vi "test_read-nmea-data2.vi"() -> ()   [LabVIEW 2019] (continued)
F9P\t$GNRMC,060930.00,A,3723.60323,N,12656.90330,E,1.432,,250720,,,A,V*10\n\t\n15:09:28.28\tF9P\t$GNVTG,,T,,M,1.432,N,2.653,K,A*3B\n\t\n15:09:28.30\tF9P\t$GNGGA,060930.00,3723.60323,N,12656.90330,E,1,12,0.66,57.5,M,18.5,M,,*78\n\t\n15:09:28.32\tF9P\t$GNGSA,A,3,12,06,19,05,17,09,04,02,,,,,1.21,0.66,1.01,1*02\n\t\n15:09:28.34\tF9P\t$GNGSA,A,3,85,71,84,,,,,,,,,,1.21,0.66,1.01,2*07\n\t\n15:09:28.36\tF9P\t$GNGSA,A,3,36,19,11,04,09,12,,,,,,,1.21,0.66,1.01,3*02\n\t\n15:09:28.38\tF9P\t$GNGSA,A,3,14,11,33,,,,,,,,,,1.21,0.66,1.01,4*03\n\t\n15:09:28.40\tF9P\t$GPGSV,3,1,09,02,54,318,30,04,19,044,21,05,36,246,27,06,65,046,24,1*6E\n\t\n15:09:28.42\tF9P\t$GPGSV,3,2,09,09,45,075,32,12,24,278,25,17,34,153,23,19,53,156,24,1*65\n\t\n15:09:28.44\tF9P\t$GPGSV,3,3,09,25,12,307,23,1*5C\n\t\n15:09:28.46\tF9P\t$GPGSV,3,1,09,02,54,318,,04,19,044,14,05,36,246,18,06,65,046,20,6*64\n\t\n15:09:28.48\tF9P\t$GPGSV,3,2,09,09,45,075,20,12,24,278,16,17,34,153,,19,53,156,,6*66\n\t\n15:09:28.50\tF9P\t$GPGSV,3,3,09,25,12,307,,6*5A\n\t\n15:09:28.52\tF9P\t$GLGSV,2,1,08,69,13,031,,70,73,042,,71,50,204,25,72,03,209,,1*76\n\t\n15:09:28.54\tF9P\t$GLGSV,2,2,08,77,01,327,,84,21,121,12,85,70,063,23,86,35,329,,1*77\n\t\n15:09:28.56\tF9P\t$GLGSV,2,1,08,69,13,031,15,70,73,042,,71,50,204,22,72,03,209,,3*77\n\t\n15:09:28.58\tF9P\t$GLGSV,2,2,08,77,01,327,,84,21,121,17,85,70,063,21,86,35,329,,3*72\n\t\n15:09:28.60\tF9P\t$GAGSV,2,1,08,02,09,298,21,04,65,120,25,09,30,193,17,11,70,356,22,7*70\n\t\n15:09:28.62\tF9P\t$GAGSV,2,2,08,12,41,101,19,19,27,046,10,25,10,250,,36,25,307,28,7*76\n\t\n15:09:28.64\tF9P\t$GAGSV,2,1,08,02,09,298,,04,65,120,26,09,30,193,,11,70,356,19,2*7B\n\t\n15:09:28.66\tF9P\t$GAGSV,2,2,08,12,41,101,,19,27,046,,25,10,250,,36,25,307,23,2*71\n\t\n15:09:28.68\tF9P\t$GBGSV,1,1,03,11,51,130,12,14,86,148,17,33,59,218,21,1*44\n\t\n15:09:28.70\tF9P\t$GBGSV,1,1,04,08,,,21,11,51,130,23,14,86,148,30,33,59,218,,3*4E\n\t\n15:09:28.72\tF9P\t$GNGLL,3723.60323,N,12656.90330,E,060930.00,A,A*75\n\t\n15:09:28.74\tF9P\t\t\n15:09:28.76\tF9P\t\t\n15:09:28.78\tF9P\t\t\n15:09:28.80\tF9P\t\t\n15:09:28.82\tF9P\t\t\n15:09:28.84\tF9P\t\t\n15:09:28.86\tF9P\t\t\n15:09:28.88\tF9P\t\t\n15:09:28.90\tF9P\t\t\n15:09:28.92\tF9P\t\t\n15:09:28.94\tF9P\t\t\n15:09:28.96\tF9P\t\t\n15:09:28.98\tF9P\t\t\n15:09:29.00\tF9P\t\t\n15:09:29.02\tF9P\t\t\n15:09:29.04\tF9P\t\t\n15:09:29.06\tF9P\t\t\n15:09:29.08\tF9P\t\t\n15:09:29.10\tF9P\t\t\n15:09:29.12\tF9P\t\t\n15:09:29.14\tF9P\t\t\n15:09:29.16\tF9P\t\t\n15:09:29.18\tF9P\t\t\n15:09:29.20\tF9P\t\t\n15:09:29.22\tF9P\t\t\n15:09:29.24\tF9P\t$GNRMC,060931.00,A,3723.60267,N,12656.90271,E,2.484,237.32,250720,,,A,V*03\n\t\n15:09:29.26\tF9P\t$GNVTG,237.32,T,,M,2.484,N,4.600,K,A*2C\n\t\n15:09:29.28\tF9P\t$GNGGA,060931.00,3723.60267,N,12656.90271,E,1,12,0.67,56.1,M,18.5,M,,*78\n\t\n15:09:29.30\tF9P\t$GNGSA,A,3,12,06,19,05,17,09,04,02,,,,,1.23,0.67,1.03,1*03\n\t\n15:09:29.32\tF9P\t$GNGSA,A,3,85,71,84,,,,,,,,,,1.23,0.67,1.03,2*06\n\t\n15:09:29.34\tF9P\t$GNGSA,A,3,36,19,11,04,09,12,,,,,,,1.23,0.67,1.03,3*03\n\t\n15:09:29.36\tF9P\t$GNGSA,A,3,14,11,33,,,,,,,,,,1.23,0.67,1.03,4*02\n\t\n15:09:29.38\tF9P\t$GPGSV,3,1,09,02,54,318,24,04,19,044,19,05,36,246,33,06,65,046,23,1*62\n\t\n15:09:29.40\tF9P\t$GPGSV,3,2,09,09,45,075,24,12,24,278,24,17,34,153,30,19,53,156,23,1*66\n\t\n15:09:29.42\tF9P\t$GPGSV,3,3,09,25,12,307,23,1*5C\n\t\n15:09:29.44\tF9P\t$GPGSV,3,1,09,02,54,318,,04,19,044,14,05,36,246,16,06,65,046,21,6*6B\n\t\n15:09:29.46\tF9P\t$GPGSV,3,2,09,09,45,075,18,12,24,278,17,17,34,153,,19,53,156,,6*6C\n\t\n15:09:29.48\tF9P\t$GPGSV,3,3,09,25,12,307,,6*5A\n\t\n15:09:29.50\tF9P\t$GLGSV,2,1,08,69,13,031,,70,73,042,,71,50,204,32,72,03,209,,1*70\n\t\n15:09:29.52\tF9P\t$GLGSV,2,2,08,77,01,327,,84,21,121,13,85,70,063,24,86,35,329,,1*71\n\t\n15:09:29.54\tF9P\t$GLGSV,2,1,08,69,13,031,,70,73,042,,71,50,204,23,72,03,209,,3*72\n\t\n15:09:29.56\tF9P\t$GLGSV,2,2,08,77,01,327,,84,21,121,16,85,70,063,20,86,35,329,,3*72\n\t\n15:09:29.58\tF9P\t$GAGSV,2,1,08,02,09,298,17,04,65,120,24,09,30,193,16,11,70,356,23,7*74\n\t\n15:09:29.60\tF9P\t$GAGSV,2,2,08,12,41,101,17,19,27,046,14,25,10,250,,36,25,307,32,7*77\n\t\n15:09:29.62\tF9P\t$GAGSV,2,1,08,02,09,298,,04,65,120,27,09,30,193,,11,70,356,19,2*7A\n\t\n15:09:29.64\tF9P\t$GAGSV,2,2,08,12,41,101,,19,27,046,,25,10,250,,36,25,307,23,2*71\n\t\n15:09:29.66\tF9P\t$GBGSV,1,1,03,11,51,130,07,14,86,148,10,33,59,218,17,1*42\n\t\n15:09:29.68\tF9P\t$GBGSV,1,1,04,08,,,20,11,51,130,21,14,86,148,29,33,59,218,,3*45\n\t\n15:09:29.70\tF9P\t$GNGLL,3723.60267,N,12656.90271,E,060931.00,A,A*71\n\t\n15:09:29.72\tF9P\t\t\n15:09:29.74\tF9P\t\t\n15:09:29.76\tF9P\t\t\n15:09:29.78\tF9P\t\t\n15:09:29.80\tF9P\t\t\n15:09:29.82\tF9P\t\t\n15:09:29.84\tF9P\t\t\n15:09:29.86\tF9P\t\t\n15:09:29.88\tF9P\t\t\n15:09:29.90\tF9P\t\t\n15:09:29.92\tF9P\t\t\n15:09:29.94\tF9P\t\t\n15:09:29.96\tF9P\t\t\n15:09:29.98\tF9P\t\t\n15:09:30.00\tF9P\t\t\n15:09:30.02\tF9P\t\t\n15:09:30.05\tF9P\t\t\n15:09:30.07\tF9P\t\t\n15:09:30.09\tF9P\t\t\n15:09:30.11\tF9P\t\t\n15:09:30.13\tF9P\t\t\n15:09:30.15\tF9P\t\t\n15:09:30.17\tF9P\t\t\n15:09:30.19\tF9P\t\t\n15:09:30.21\tF9P\t\t\n15:09:30.23\tF9P\t\t\n15:09:30.25\tF9P\t$GNRMC,060932.00,A,3723.60237,N,12656.90214,E,1.383,237.05,250720,,,A,V*01\n\t\n15:09:30.27\tF9P\t$GNVTG,237.05,T,,M,1.383,N,2.562,K,A*2A\n\t\n15:09:30.29\tF9P\t$GNGGA,060932.00,3723.60237,N,12656.90214,E,1,12,0.67,55.8,M,18.5,M,,*77\n\t\n15:09:30.31\tF9P\t$GNGSA,A,3,12,06,19,05,17,09,04,02,,,,,1.23,0.67,1.03,1*03\n\t\n15:09:30.33\tF9P\t$GNGSA,A,3,85,71,84,,,,,,,,,,1.23,0.67,1.03,2*06\n\t\n15:09:30.35\tF9P\t$GNGSA,A,3,36,19,11,04,09,12,,,,,,,1.23,0.67,1.03,3*03\n\t\n15:09:30.37\tF9P\t$GNGSA,A,3,14,11,,,,,,,,,,,1.23,0.67,1.03,4*02\n\t\n15:09:30.39\tF9P\t$GPGSV,3,1,09,02,54,318,31,04,19,044,17,05,36,246,29,06,65,046,29,1*69\n\t\n15:09:30.41\tF9P\t$GPGSV,3,2,09,09,45,075,28,12,24,278,23,17,34,153,24,19,53,156,33,1*69\n\t\n15:09:30.43\tF9P\t$GPGSV,3,3,09,25,12,307,24,1*5B\n\t\n15:09:30.45\tF9P\t$GPGSV,3,1,09,02,54,318,,04,19,044,12,05,36,246,17,06,65,046,20,6*6D\n\t\n15:09:30.47\tF9P\t$GPGSV,3,2,09,09,45,075,17,12,24,278,16,17,34,153,,19,53,156,,6*62\n\t\n15:09:30.49\tF9P\t$GPGSV,3,3,09,25,12,307,,6*5A\n\t\n15:09:30.51\tF9P\t$GLGSV,2,1,08,69,13,031,,70,73,042,,71,50,204,30,72,03,209,,1*72\n\t\n15:09:30.53\tF9P\t$GLGSV,2,2,08,77,01,327,,84,21,121,12,85,70,063,30,86,35,329,,1*75\n\t\n15:09:30.55\tF9P\t$GLGSV,2,1,08,69,13,031,,70,73,042,,71,50,204,24,72,03,209,,3*75\n\t\n15:09:30.57\tF9P\t$GLGSV,2,2,08,77,01,327,,84,21,121,17,85,70,063,19,86,35,329,,3*79\n\t\n15:09:30.59\tF9P\t$GAGSV,2,1,08,02,09,298,16,04,65,120,24,09,30,193,16,11,70,356,23,7*75\n\t\n15:09:30.61\tF9P\t$GAGSV,2,2,08,12,41,101,16,19,27,046,13,25,10,250,,36,25,307,29,7*7B\n\t\n15:09:30.63\tF9P\t$GAGSV,2,1,08,02,09,298,,04,65,120,27,09,30,193,,11,70,356,21,2*71\n\t\n15:09:30.65\tF9P\t$GAGSV,2,2,08,12,41,101,,19,27,046,,25,10,250,,36,25,307,25,2*77\n\t\n15:09:30.67\tF9P\t$GBGSV,1,1,03,11,51,130,,14,86,148,07,33,59,218,,1*45\n\t\n15:09:30.69\tF9P\t$GBGSV,1,1,04,08,,,18,11,51,130,21,14,86,148,32,33,59,218,,3*44\n\t\n15:09:30.71\tF9P\t$GNGLL,3723.60237,N,12656.90214,E,060932.00,A,A*74\n\t\n15:09:30.73\tF9P\t\t\n15:09:30.75\tF9P\t\t\n15:09:30.77\tF9P\t\t\n15:09:30.79\tF9P\t\t\n15:09:30.81\tF9P\t\t\n15:09:30.83\tF9P\t\t\n15:09:30.85\tF9P\t\t\n15:09:30.87\tF9P\t\t\n15:09:30.89\tF9P\t\t\n15:09:30.91\tF9P\t\t\n15:09:30.93\tF9P\t\t\n15:09:30.95\tF9P\t\t\n15:09:30.97\tF9P\t\t\n15:09:30.99\tF9P\t\t\n15:09:31.01\tF9P\t\t\n15:09:31.03\tF9P\t\t\n15:09:31.05\tF9P\t\t\n15:09:31.07\tF9P\t\t\n15:09:31.09\tF9P\t\t\n15:09:31.11\tF9P\t\t\n15:09:31.13\tF9P\t\t\n15:09:31.15\tF9P\t\t\n15:09:31.17\tF9P\t\t\n15:09:31.19\tF9P\t\t\n15:09:31.21\tF9P\t\t\n15:09:31.23\tF9P\t\t\n15:09:31.25\tF9P\t$GNRMC,060933.00,A,3723.60178,N,12656.90204,E,1.526,218.15,250720,,,A,V*0C\n\t\n15:09:31.27\tF9P\t$GNVTG,218.15,T,,M,1.526,N,2.826,K,A*22\n\t\n15:09:31.29\tF9P\t$GNGGA,060933.00,3723.60178,N,12656.90204,E,1,12,0.69,54.6,M,18.5,M,,*7E\n\t\n15:09:31.31\tF9P\t$GNGSA,A,3,12,06,19,05,17,09,02,,,,,,1.30,0.69,1.11,1*08\n\t\n15:09:31.33\tF9P\t$GNGSA,A,3,85,71,84,,,,,,,,,,1.30,0.69,1.11,2*09\n\t\n15:09:31.35\tF9P\t$GNGSA,A,3,36,19,11,04,09,12,,,,,,,1.30,0.69,1.11,3*0C\n\t\n15:09:31.37\tF9P\t$GNGSA,A,3,14,11,,,,,,,,,,,1.30,0.69,1.11,4*0D\n\t\n15:09:31.39\tF9P\t$GPGSV,3,1,09,02,54,318,30,04,19,044,,05,36,246,27,06,65,046,27,1*6E\n\t\n15:09:31.41\tF9P\t$GPGSV,3,2,09,09,45,075,28,12,24,278,27,17,34,153,30,19,53,156,32,1*69\n\t\n15:09:31.43\tF9P\t$GPGSV,3,3,09,25,12,307,27,1*58\n\t\n15:09:31.45\tF9P\t$GPGSV,3,1,09,02,54,318,,04,19,044,13,05,36,246,19,06,65,046,20,6*62\n\t\n15:09:31.47\tF9P\t$GPGSV,3,2,09,09,45,075,17,12,24,278,15,17,34,153,,19,53,156,,6*61\n\t\n15:09:31.49\tF9P\t$GPGSV,3,3,09,25,12,307,,6*5A\n\t\n15:09:31.51\tF9P\t$GLGSV,2,1,08,69,13,031,,70,73,042,,71,50,204,29,72,03,209,,1*7A\n\t\n15:09:31.53\tF9P\t$GLGSV,2,2,08,77,01,327,,84,21,121,12,85,70,063,30,86,35,329,,1*75\n\t\n15:09:31.55\tF9P\t$GLGSV,2,1,08,69,13,031,,70,73,042,,71,50,204,25,72,03,209,,3*74\n\t\n15:09:31.57\tF9P\t$GLGSV,2,2,08,77,01,327,,84,21,121,19,85,70,063,19,86,35,329,,3*77\n\t\n15:09:31.59\tF9P\t$GAGSV,2,1,08,02,09,298,15,04,65,120,29,09,30,193,14,11,70,356,22,7*78\n\t\n15:09:31.61\tF9P\t$GAGSV,2,2,08,12,41,101,17,19,27,046,11,25,10,250,,36,25,307,32,7*72\n\t\n15:09:31.63\tF9P\t$GAGSV,2,1,08,02,09,298,,04,65,120,27,09,30,193,,11,70,356,22,2*72\n\t\n15:09:31.65\tF9P\t$GAGSV,2,2,08,12,41,101,,19,27,046,,25,10,250,,36,25,307,30,2*73\n\t\n15:09:31.67\tF9P\t$GBGSV,1,1,04,07,,,21,11,51,130,,14,86,148,18,33,59,218,25,1*4F\n\t\n15:09:31.69\tF9P\t$GBGSV,1,1,04,08,,,27,11,51,130,21,14,86,148,32,33,59,218,,3*48\n\t\n15:09:31.71\tF9P\t$GNGLL,3723.60178,N,12656.90204,E,060933.00,A,A*7C\n\t\n15:09:31.73\tF9P\t\t\n15:09:31.75\tF9P\t\t\n15:09:31.77\tF9P\t\t\n15:09:31.79\tF9P\t\t\n15:09:31.81\tF9P\t\t\n15:09:31.83\tF9P\t\t\n15:09:31.85\tF9P\t\t\n15:09:31.87\tF9P\t\t\n15:09:31.89\tF9P\t\t\n15:09:31.91\tF9P\t\t\n15:09:31.93\tF9P\t\t\n15:09:31.95\tF9P\t\t\n15:09:31.97\tF9P\t\t\n15:09:31.99\tF9P\t\t\n15:09:32.01\tF9P\t\t\n15:09:32.03\tF9P\t\t\n15:09:32.05\tF9P\t\t\n15:09:32.07\tF9P\t\t\n15:09:32.09\tF9P\t\t\n15:09:32.11\tF9P\t\t\n15:09:32.13\tF9P\t\t\n15:09:32.15\tF9P\t\t\n15:09:32.17\tF9P\t\t\n15:09:32.19\tF9P\t\t\n15:09:32.21\tF9P\t\t\n15:09:32.23\tF9P\t\t\n15:09:32.25\tF9P\t$GNRMC,060934.00,A,3723.60110,N,12656.90170,E,1.480,224.53,250720,,,A,V*05\n\t\n15:09:32.27\tF9P\t$GNVTG,224.53,T,,M,1.480,N,2.741,K,A*2C\n\t\n15:09:32.29\tF9P\t$GNGGA,060934.00,3723.60110,N,12656.90170,E,1,12,0.68,54.6,M,18.5,M,,*76\n\t\n15:09:32.31\tF9P\t$GNGSA,A,3,12,06,19,05,17,09,04,02,,,,,1.31,0.68,1.12,1*0F\n\t\n15:09:32.33\tF9P\t$GNGSA,A,3,85,71,84,,,,,,,,,,1.31,0.68,1.12,2*0A\n\t\n15:09:32.35\tF9P\t$GNGSA,A,3,36,19,11,04,09,12,,,,,,,1.31,0.68,1.12,3*0F\n\t\n15:09:32.37\tF9P\t$GNGSA,A,3,14,11,33,,,,,,,,,,1.31,0.68,1.12,4*0E\n\t\n15:09:32.39\tF9P\t$GPGSV,3,1,09,02,54,318,34,04,19,044,20,05,36,246,31,06,65,046,27,1*6F\n\t\n15:09:32.41\tF9P\t$GPGSV,3,2,09,09,45,075,32,12,24,278,26,17,34,153,32,19,53,156,27,1*65\n\t\n15:09:32.43\tF9P\t$GPGSV,3,3,09,25,12,307,26,1*59\n\t\n15:09:32.45\tF9P\t$GPGSV,3,1,09,02,54,318,,04,19,044,12,05,36,246,20,06,65,046,21,6*68\n\t\n15:09:32.47\tF9P\t$GPGSV,3,2,09,09,45,075,18,12,24,278,15,17,34,153,,19,53,156,,6*6E\n\t\n15:09:32.49\tF9P\t$GPGSV,3,3,09,25,12,307,,6*5A\n\t\n15:09:32.51\tF9P\t$GLGSV,2,1,08,69,13,031,,70,73,042,,71,50,204,33,72,03,209,,1*71\n\t\n15:09:32.53\tF9P\t$GLGSV,2,2,08,77,01,327,,84,21,121,12,85,70,063,29,86,35,329,,1*7D\n\t\n15:09:32.55\tF9P\t$GLGSV,2,1,08,69,13,031,,70,73,042,,71,50,204,25,72,03,209,,3*74\n\t\n15:09:32.57\tF9P\t$GLGSV,2,2,08,77,01,327,,84,21,121,18,85,70,063,19,86,35,329,,3*76\n\t\n15:09:32.59\tF9P\t$GAGSV,2,1,08,02,09,298,15,04,65,120,30,09,30,193,16,11,70,356,22,7*72\n\t\n15:09:32.61\tF9P\t$GAGSV,2,2,08,12,41,101,17,19,27,046,11,25,10,250,,36,25,307,26,7*77\n\t\n15:09:32.63\tF9P\t$GAGSV,2,1,08,02,09,298,,04,65,120,25,09,30,193,,11,70,356,22,2*70\n\t\n15:09:32.65\tF9P\t$GAGSV,2,2,08,12,41,101,,19,27,046,,25,10,250,,36,25,307,23,2*71\n\t\n15:09:32.67\tF9P\t$GBGSV,2,1,06,06,,,23,07,,,28,08,,,27,11,51,130,12,1*41\n\t\n15:09:32.69\tF9P\t$GBGSV,2,2,06,14,86,148,18,33,59,218,33,1*78\n\t\n15:09:32.71\tF9P\t$GBGSV,1,1,04,08,,,27,11,51,130,21,14,86,148,26,33,59,218,,3*4D\n\t\n15:09:32.73\tF9P\t$GNGLL,3723.60110,N,12656.90170,E,060934.00,A,A*75\n\t\n15:09:32.75\tF9P\t\t\n15:09:32.77\tF9P\t\t\n15:09:32.79\tF9P\t\t\n15:09:32.81\tF9P\t\t\n15:09:32.83\tF9P\t\t\n15:09:32.85\tF9P\t\t\n15:09:32.87\tF9P\t\t\n15:09:32.89\tF9P\t\t\n15:09:32.91\tF9P\t\t\n15:09:32.93\tF9P\t\t\n15:09:32.95\tF9P\t\t\n15:09:32.97\tF9P\t\t\n15:09:32.99\tF9P\t\t\n15:09:33.01\tF9P\t\t\n15:09:33.03\tF9P\t\t\n15:09:33.05\tF9P\t\t\n15:09:33.07\tF9P\t\t\n15:09:33.09\tF9P\t\t\n15:09:33.11\tF9P\t\t\n15:09:33.13\tF9P\t\t\n15:09:33.15\tF9P\t\t\n15:09:33.17\tF9P\t\t\n15:09:33.19\tF9P\t\t\n15:09:33.21\tF9P\t\t\n15:09:33.23\tF9P\t\t\n15:09:33.25\tF9P\t$GNRMC,060935.00,A,3723.60013,N,12656.90147,E,2.238,224.68,250720,,,A,V*0C\n\t\n15:09:33.27\tF9P\t$GNVTG,224.68,T,,M,2.238,N,4.145,K,A*26\n\t\n15:09:33.29\tF9P\t$GNGGA,060935.00,3723.60013,N,12656.90147,E,1,12,0.64,52.8,M,18.5,M,,*75\n\t\n15:09:33.31\tF9P\t$GNGSA,A,3,12,06,19,05,17,09,04,02,,,,,1.19,0.64,1.00,1*0A\n\t\n15:09:33.33\tF9P\t$GNGSA,A,3,85,71,84,,,,,,,,,,1.19,0.64,1.00,2*0F\n\t\n15:09:33.35\tF9P\t$GNGSA,A,3,36,19,11,04,09,12,,,,,,,1.19,0.64,1.00,3*0A\n\t\n15:09:33.37\tF9P\t$GNGSA,A,3,14,11,33,,,,,,,,,,1.19,0.64,1.00,4*0B\n\t\n15:09:33.39\tF9P\t$GPGSV,3,1,09,02,54,318,28,04,19,044,20,05,36,246,28,06,65,046,32,1*6E\n\t\n15:09:33.41\tF9P\t$GPGSV,3,2,09,09,45,075,32,12,24,278,24,17,34,153,34,19,53,156,34,1*63\n\t\n15:09:33.43\tF9P\t$GPGSV,3,3,09,25,12,307,25,1*5A\n\t\n15:09:33.45\tF9P\t$GPGSV,3,1,09,02,54,318,,04,19,044,12,05,36,246,19,06,65,046,21,6*62\n\t\n15:09:33.47\tF9P\t$GPGSV,3,2,09,09,45,075,21,12,24,278,13,17,34,153,21,19,53,156,,6*61\n\t\n15:09:33.49\tF9P\t$GPGSV,3,3,09,25,12,307,,6*5A\n\t\n15:09:33.51\tF9P\t$GLGSV,2,1,08,69,13,031,,70,73,042,,71,50,204,29,72,03,209,,1*7A\n\t\n15:09:33.53\tF9P\t$GLGSV,2,2,08,77,01,327,,84,21,121,10,85,70,063,27,86,35,329,,1*71\n\t\n15:09:33.55\tF9P\t$GLGSV,2,1,08,69,13,031,,70,73,042,,71,50,204,26,72,03,209,,3*77\n\t\n15:09:33.57\tF9P\t$GLGSV,2,2,08,77,01,327,,84,21,121,19,85,70,063,19,86,35,329,,3*77\n\t\n15:09:33.59\tF9P\t$GAGSV,2,1,08,02,09,298,12,04,66,119,28,09,30,193,16,11,70,356,23,7*74\n\t\n15:09:33.61\tF9P\t$GAGSV,2,2,08,12,41,101,17,19,27,046,10,25,10,250,,36,25,307,29,7*79\n\t\n15:09:33.63\tF9P\t$GAGSV,2,1,08,02,09,298,,04,66,119,24,09,30,193,,11,70,356,21,2*7B\n\t\n15:09:33.65\tF9P\t$GAGSV,2,2,08,12,41,101,,19,27,046,,25,10,250,,36,25,307,22,2*70\n\t\n15:09:33.67\tF9P\t$GBGSV,2,1,06,06,,,25,07,,,25,08,,,25,11,51,130,13,1*49\n\t\n15:09:33.69\tF9P\t$GBGSV,2,2,06,14,86,148,27,33,59,218,25,1*73\n\t\n15:09:33.71\tF9P\t$GBGSV,1,1,04,08,,,26,11,51,130,22,14,86,148,31,33,59,218,,3*49\n\t\n15:09:33.73\tF9P\t$GNGLL,3723.60013,N,12656.90147,E,060935.00,A,A*72\n\t\n15:09:33.75\tF9P\t\t\n15:09:33.77\tF9P\t\t\n15:09:33.79\tF9P\t\t\n15:09:33.81\tF9P\t\t\n15:09:33.83\tF9P\t\t\n15:09:33.85\tF9P\t\t\n15:09:33.87\tF9P\t\t\n15:09:33.89\tF9P\t\t\n15:09:33.91\tF9P\t\t\n15:09:33.93\tF9P\t\t\n15:09:33.95\tF9P\t\t\n15:09:33.97\tF9P\t\t\n15:09:33.99\tF9P\t\t\n15:09:34.01\tF9P\t\t\n15:09:34.03\tF9P\t\t\n15:09:34.05\tF9P\t\t\n15:09:34.07\tF9P\t\t\n15:09:34.09\tF9P\t\t\n15:09:34.11\tF9P\t\t\n15:09:34.13\tF9P\t\t\n15:09:34.15\tF9P\t\t\n15:09:34.17\tF9P\t\t\n15:09:34.19\tF9P\t\t\n15:09:34.21\tF9P\t\t\n15:09:34.23\tF9P\t\t\n15:09:34.25\tF9P\t$GNRMC,060936.00,A,3723.59866,N,12656.90154,E,2.355,237.67,250720,,,A,V*0A\n\t\n15:09:34.27\tF9P\t$GNVTG,237.67,T,,M,2.355,N,4.361,K,A*25\n\t\n15:09:34.29\tF9P\t$GNGGA,060936.00,3723.59866,N,12656.90154,E,1,12,0.64,49.6,M,18.5,M,,*70\n\t\n15:09:34.31\tF9P\t$GNGSA,A,3,12,06,19,05,17,09,04,02,,,,,1.19,0.64,1.00,1*0A\n\t\n15:09:34.33\tF9P\t$GNGSA,A,3,85,71,84,,,,,,,,,,1.19,0.64,1.00,2*0F\n\t\n15:09:34.35\tF9P\t$GNGSA,A,3,36,19,11,04,09,12,,,,,,,1.19,0.64,1.00,3*0A\n\t\n15:09:34.37\tF9P\t$GNGSA,A,3,14,11,33,,,,,,,,,,1.19,0.64,1.00,4*0B\n\t\n15:09:34.39\tF9P\t$GPGSV,3,1,09,02,54,318,27,04,19,044,17,05,36,246,32,06,65,046,31,1*6D\n\t\n15:09:34.41\tF9P\t$GPGSV,3,2,09,09,45,075,35,12,24,278,21,17,34,153,39,19,53,156,31,1*69\n\t\n15:09:34.43\tF9P\t$GPGSV,3,3,09,25,12,307,22,1*5D\n\t\n15:09:34.45\tF9P\t$GPGSV,3,1,09,02,54,318,,04,19,044,13,05,36,246,18,06,65,046,22,6*61\n\t\n15:09:34.47\tF9P\t$GPGSV,3,2,09,09,45,075,22,12,24,278,13,17,34,153,22,19,53,156,,6*61\n\t\n15:09:34.49\tF9P\t$GPGSV,3,3,09,25,12,307,,6*5A\n\t\n15:09:34.51\tF9P\t$GLGSV,2,1,08,69,13,031,,70,73,042,,71,50,204,28,72,03,209,,1*7B\n\t\n15:09:34.53\tF9P\t$GLGSV,2,2,08,77,01,327,,84,21,121,09,85,70,063,26,86,35,329,,1*78\n\t\n15:09:34.55\tF9P\t$GLGSV,2,1,08,69,13,031,,70,73,042,,71,50,204,24,72,03,209,,3*75\n\t\n15:09:34.57\tF9P\t$GLGSV,2,2,08,77,01,327,,84,21,121,18,85,70,063,19,86,35,329,,3*76\n\t\n15:09:34.59\tF9P\t$GAGSV,2,1,08,02,09,298,12,04,66,119,32,09,30,193,20,11,70,356,24,7*7D\n\t\n15:09:34.61\tF9P\t$GAGSV,2,2,08,12,41,101,16,19,27,046,09,25,10,250,,36,25,307,29,7*70\n\t\n15:09:34.63\tF9P\t$GAGSV,2,1,08,02,09,298,,04,66,119,24,09,30,193,22,11,70,356,19,2*70\n\t\n15:09:34.65\tF9P\t$GAGSV,2,2,08,12,41,101,,19,27,046,,25,10,250,,36,25,307,23,2*71\n\t\n15:09:34.67\tF9P\t$GBGSV,1,1,03,11,51,130,15,14,86,148,28,33,59,218,25,1*4B\n\t\n15:09:34.69\tF9P\t$GBGSV,1,1,04,08,,,24,11,51,130,22,14,86,148,30,33,59,218,,3*4A\n\t\n15:09:34.71\tF9P\t$GNGLL,3723.59866,N,12656.90154,E,060936.00,A,A*73\n\t\n15:09:34.73\tF9P\t\t\n15:09:34.75\tF9P\t\t\n15:09:34.77\tF9P\t\t\n15:09:34.79\tF9P\t\t\n15:09:34.81\tF9P\t\t\n15:09:34.83\tF9P\t\t\n15:09:34.85\tF9P\t\t\n15:09:34.87\tF9P\t\t\n15:09:34.89\tF9P\t\t\n15:09:34.91\tF9P\t\t\n15:09:34.93\tF9P\t\t\n15:09:34.95\tF9P\t\t\n15:09:34.97\tF9P\t\t\n15:09:34.99\tF9P\t\t\n15:09:35.01\tF9P\t\t\n15:09:35.03\tF9P\t\t\n15:09:35.05\tF9P\t\t\n15:09:35.07\tF9P\t\t\n15:09:35.09\tF9P\t\t\n15:09:35.11\tF9P\t\t\n15:09:35.13\tF9P\t\t\n15:09:35.15\tF9P\t\t\n15:09:35.17\tF9P\t\t\n15:09:35.19\tF9P\t\t\n15:09:35.21\tF9P\t\t\n15:09:35.23\tF9P\t\t\n15:09:35.25\tF9P\t$GNRMC,060937.00,A,3723.59722,N,12656.90157,E,2.229,233.59,250720,,,A,V*04\n\t\n15:09:35.27\tF9P\t$GNVTG,233.59,T,,M,2.229,N,4.128,K,A*29\n\t\n15:09:35.29\tF9P\t$GNGGA,060937.00,3723.59722,N,12656.90157,E,1,12,0.67,47.2,M,18.5,M,,*74\n\t\n15:09:35.31\tF9P\t$GNGSA,A,3,12,06,19,05,17,09,04,02,,,,,1.29,0.67,1.10,1*0B\n\t\n15:09:35.33\tF9P\t$GNGSA,A,3,85,71,84,,,,,,,,,,1.29,0.67,1.10,2*0E\n\t\n15:09:35.35\tF9P\t$GNGSA,A,3,36,19,11,04,09,12,,,,,,,1.29,0.67,1.10,3*0B\n\t\n15:09:35.37\tF9P\t$GNGSA,A,3,14,11,33,,,,,,,,,,1.29,0.67,1.10,4*0A\n\t\n15:09:35.39\tF9P\t$GPGSV,3,1,09,02,54,318,28,04,19,044,17,05,36,246,28,06,65,046,29,1*60\n\t\n15:09:35.41\tF9P\t$GPGSV,3,2,09,09,45,075,30,12,24,278,20,17,34,153,38,19,53,156,32,1*6F\n\t\n15:09:35.43\tF9P\t$GPGSV,3,3,09,25,12,307,22,1*5D\n\t\n15:09:35.45\tF9P\t$GPGSV,3,1,09,02,54,318,,04,19,044,10,05,36,246,20,06,65,046,24,6*6F\n\t\n15:09:35.47\tF9P\t$GPGSV,3,2,09,09,45,075,22,12,24,278,,17,34,153,24,19,53,156,,6*65\n\t\n15:09:35.49\tF9P\t$GPGSV,3,3,09,25,12,307,,6*5A\n\t\n15:09:35.51\tF9P\t$GLGSV,2,1,08,69,13,031,,70,73,042,,71,50,204,28,72,03,209,,1*7B\n\t\n15:09:35.53\tF9P\t$GLGSV,2,2,08,77,01,327,,84,21,121,08,85,70,063,27,86,35,329,,1*78\n\t\n15:09:35.55\tF9P\t$GLGSV,2,1,08,69,13,031,,70,73,042,,71,50,204,22,72,03,209,,3*73\n\t\n15:09:35.57\tF9P\t$GLGSV,2,2,08,77,01,327,,84,21,121,15,85,70,063,19,86,35,329,,3*7B\n\t\n15:09:35.59\tF9P\t$GAGSV,2,1,08,02,09,298,15,04,66,119,33,09,30,193,22,11,70,356,26,7*7B\n\t\n15:09:35.61\tF9P\t$GAGSV,2,2,08,12,41,101,19,19,27,046,12,25,10,250,,36,25,307,29,7*75\n\t\n15:09:35.63\tF9P\t$GAGSV,2,1,08,02,09,298,,04,66,119,26,09,30,193,22,11,70,356,19,2*72\n\t\n15:09:35.65\tF9P\t$GAGSV,2,2,08,12,41,101,,19,27,046,,25,10,250,,36,25,307,25,2*77\n\t\n15:09:35.67\tF9P\t$GBGSV,1,1,03,11,51,130,20,14,86,148,27,33,59,218,28,1*4F\n\t\n15:09:35.69\tF9P\t$GBGSV,1,1,04,08,,,22,11,51,130,23,14,86,148,23,33,59,218,,3*4F\n\t\n15:09:35.71\tF9P\t
